vi "getDevice.vi"(8 "error in (no error)":errorcluster, 10 "Device Number":i32, 11 "DeviceFactory in":refnum<class "DeviceFactory.lvclass">) -> (0 "error out":errorcluster, 1 "AutomatedController":refnum<class "AutomatedController.lvclass">, 3 "DeviceFactory out":refnum<class "DeviceFactory.lvclass">)   [LabVIEW 2020, in "DeviceFactory.lvclass"]
uses:
  DeviceFactory.lvclass
  Devices/AutomatedController/AutomatedController.lvclass
  DeviceFactory.lvclass/DeviceFactory.ctl
  Devices/Arduino/Arduino.lvclass
  C:/Users/fflores/Documents/GitHub Projects/HAL-with-Interfaces/Devices/AutomatedController/AutomatedController.lvclass
  Accessories/Wi-Fi Shield/Wi-Fi Shield.lvclass
  C:/Users/fflores/Documents/GitHub Projects/HAL-with-Interfaces/Interfaces/Arduino Shield/Arduino Shield.lvclass
  Interfaces/Arduino Shield/Arduino Shield.lvclass
  Devices/Arduino/Arduino.lvclass/Arduino.ctl
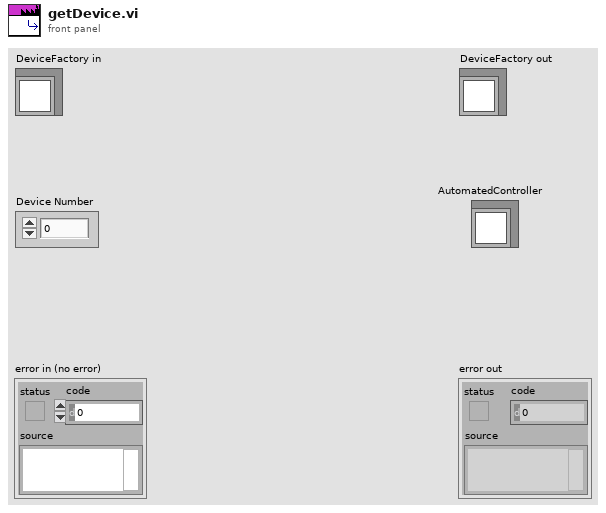
[diagram p1: front panel]
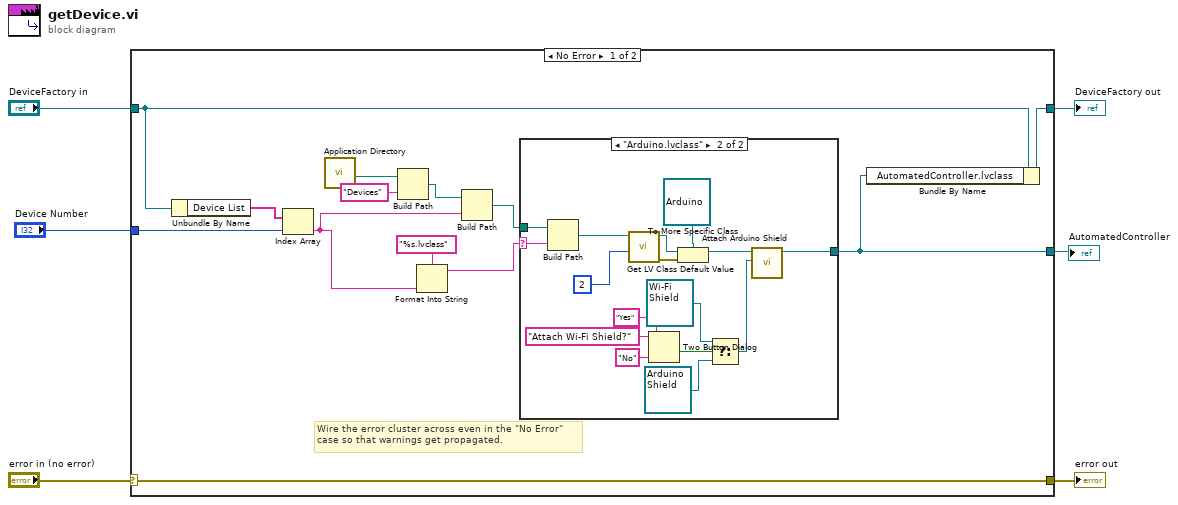
[diagram p0: block diagram]
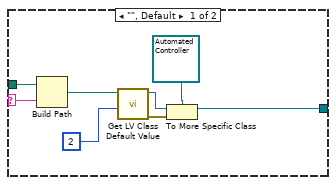
[diagram p2: hidden frame]
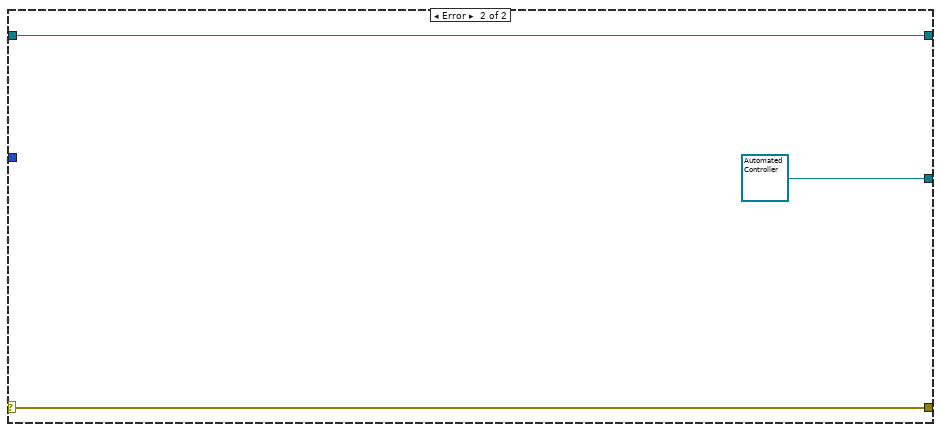
[diagram p3: hidden frame]
diagram:
  n1 = case shown="No Error" "error in (no error)" {
    selector: "error in (no error)" -> [w19 w46]
    tunnel: [w19 w46] -> w5
    tunnel: [w8 w45] -> w3
    tunnel: "DeviceFactory in" -> [w18 w45]
    tunnel: "Device Number" -> [w16 _]
    tunnel: [w7 refnum<class "AutomatedController.lvclass"> refnum ("AutomatedController.lvclass")] -> w1
    frame No Error {
      # "Wire the error cluster across even in the \"No Error\"\ncase so that warnings get propagated."
      n2 = Unbundle By Name(w18) -> ("Device List"=w17:string[])
      n3 = Index Array(array=w17, index=w16) -> (element=w10:string)
      n4 = call <vilib>:"Application Directory.vi"() -> ("Application Directory"=w15:path)
      n5 = Build Path(base path=w15, name or relative path="Devices") -> (appended path=w13:path)
      n6 = Format Into String(format string="%s.lvclass", w10) -> (resulting string=w9:string)  [unwired: 2 in, 1 out]
      n7 = Build Path(base path=w13, name or relative path=w10) -> (appended path=w12:path)
      n8 = case shown="\"Arduino.lvclass\"" w9 {
        selector: w9 -> [w26 w42]
        tunnel: w12 -> [w27 w43]
        tunnel: [w25 w35] -> w7
        frame "", Default {
          n9 = Build Path(base path=w27, name or relative path=w26) -> (appended path=w23:path)
          n10 = call <vilib>:"Get LV Class Default Value.vi"("options"=u32 2, "class path"=w23) -> ("error out"=w22:errorcluster, "object"=w20:refnum<class>)  [unwired: 8 in]
          n11 = To More Specific Class(target class=refnum<class "AutomatedController.lvclass"> refnum ("AutomatedController.lvclass"), reference=w20, error in=w22) -> (specific class reference=w25:refnum<class "AutomatedController.lvclass">)  [unwired: 1 out]
        }
        frame "Arduino.lvclass" {
          n12 = Build Path(base path=w43, name or relative path=w42) -> (appended path=w39:path)
          n13 = call <vilib>:"Get LV Class Default Value.vi"("options"=u32 2, "class path"=w39) -> ("error out"=w38:errorcluster, "object"=w36:refnum<class>)  [unwired: 8 in]
          n14 = Two Button Dialog(message="Attach Wi-Fi Shield?", 1:"No" ("F button name (\"Cancel\")"), 2:"Yes" ("T button name (\"OK\")")) -> (T button?=w31:bool)
          n15 = To More Specific Class(target class=refnum<class "Arduino.lvclass"> refnum ("Arduino.lvclass"), reference=w36, error in=w38) -> (specific class reference=w41:refnum<class "Arduino.lvclass">)  [unwired: 1 out]
          n16 = Select(t=refnum<class "Wi-Fi Shield.lvclass"> refnum ("Wi-Fi Shield.lvclass"), s=w31, f=refnum<class "Arduino Shield.lvclass"> refnum ("Arduino Shield.lvclass")) -> (s? t:f=w28:refnum<class "Arduino Shield.lvclass">)
          n17 = call "Attach Arduino Shield.vi"("Arduino Shield"=w28, "Arduino in"=w41) -> ("Arduino out"=w35:refnum<class "Arduino.lvclass">)  [unwired: 8 in, 1 out]
        }
      }
      n18 = Bundle By Name(cluster=w18, "AutomatedController.lvclass"=w7) -> (w8:refnum<class "DeviceFactory.lvclass">)
    }
    frame Error {
    }
  }
  "error out" <- w5
  "DeviceFactory out" <- w3
  "AutomatedController" <- w1
